vi "CSM - List Module Attributes.vi"(0 "CSM Name":string, 7 "Include Value? (F)":bool, 9 "Wait (5000 ms)":i32=5000, 11 "Error In":errorcluster caption="error in (no error)") -> (4 "CSM Name (Dup)":string, 6 "Attributes":string[](array[string]), 8 "Values":variant[](array[variant]), 10 "Waited (ms)":u32, 15 "error out":errorcluster)   [LabVIEW 2017, in "Communicable State Machine.lvlib"]
doc: "Lists all attribute names of the specified module. If the CSM module does not exist, this VI waits for the specified timeout duration. If the timeout is exceeded, this VI returns a timeout error.\n\n\n> [!NOTE] <b>CSM Module Attributes</b>\n>\n> CSM module attributes are a data area that can store module configuration and status, accessed by name. CSM module attributes can be used in the following scenarios:\n> - Providing a way to access and modify configuration and status information without messages. For example, a \"Connected\" attribute in a TCP module indicating whether a connection is established is more convenient to access directly.\n> - Nodes running in advanced modes, such as Worker Mode and Chain of Responsibility Mode, share the same data area, which is used for sharing data between modules.\n\n\n<b>Reference Example</b>: `[CSM-Example]\\0. Base Concepts\\6. Module Attributes.vi`.\n\n-- <b>Controls</b> --\n- <b>CSM Name</b>: CSM module name.\n- <b>Include Value? (F)</b>: Whether to include attribute values. The default is FALSE, which specifies to not include attribute values.\n- <b>Wait (5000 ms)</b>: Timeout duration for waiting module to be alive. The default is 5000 ms.\n\n-- <b>Indicators</b> --\n- <b>CSM Name (Dup)</b>: A copy of the input CSM module name.\n- <b>Attributes</b>: List of attribute names.\n- <b>Values</b>: List of attribute values.\n- <b>Waited (ms)</b>: Time elapsed while waiting."
uses:
  Communicable State Machine.lvlib
  _Support/CSMQ/_CSMOFGV(lvlibp).vi
  CSM - Wait for Module to Be Alive.vi
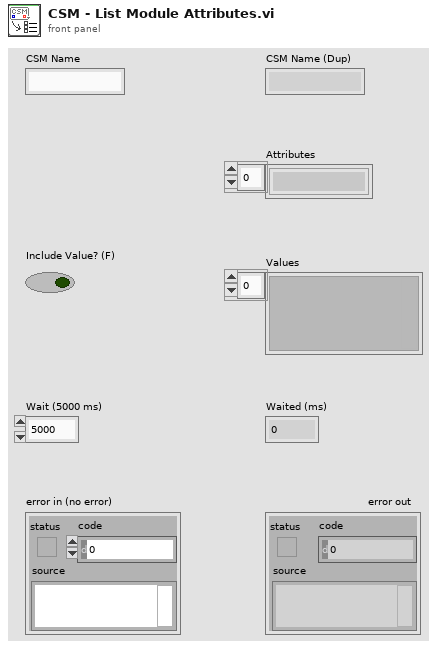
[diagram p1: front panel]
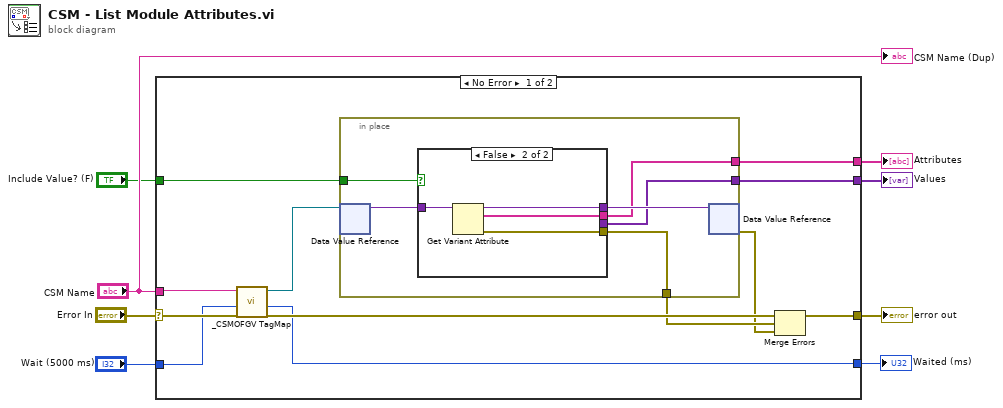
[diagram p0: block diagram]
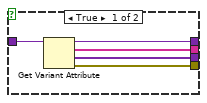
[diagram p2: hidden frame]
diagram:
  n1 = case shown="No Error" "Error In" {
    selector: "Error In" -> [w20 w36]
    tunnel: [w17 w36] -> w7
    tunnel: "CSM Name" -> [w11 _]
    tunnel: [w14 _] -> w5
    tunnel: [w13 _] -> w4
    tunnel: "Include Value? (F)" -> [w12 _]
    tunnel: "Wait (5000 ms)" -> [w10 _]
    tunnel: [w9 _] -> w1
    frame No Error {
      n2 = call "_CSMOFGV TagMap.vi"("error in (no error)"=w20, "Wait (5000 ms)"=w10, "CSM Name"=w11) -> ("error out"=w19:errorcluster, "Waited (ms)"=w9:u32, "TagMap"=w18:refnum<data-value>)  [unwired: 6 in]
      n3 = in-place {
        in-place-border: [w24] -> w16
        in-place-border: [w23] -> w14
        in-place-border: [w22] -> w13
        in-place-border: w12 -> [w21]
        n4 = in-place-dvr #1(w18) -> (w26:variant)  [unwired: 1 out]
        n5 = case shown="False" w21 {
          tunnel: w26 -> [w31 w35]
          tunnel: [w30 w34] -> w25
          tunnel: [w29 w33] -> w24
          tunnel: [w28 w32] -> w23
          tunnel: [w27 _] -> w22
          frame True {
            n6 = Get Variant Attribute(Variant=w31) -> (duplicate Variant=w30:variant, names=w28:string[], values=w27:variant[], error out=w29:errorcluster)  [unwired: 3 in]
          }
          frame False {
            n7 = Get Variant Attribute(Variant=w35) -> (duplicate Variant=w34:variant, names=w32:string[], error out=w33:errorcluster)  [unwired: 3 in, 1 out]
          }
        }
        n8 = in-place-dvr #1(w25) -> (w15:errorcluster)  [unwired: 1 out]
      }
      n9 = Merge Errors(w19, w16, w15) -> (w17:errorcluster)
    }
    frame Error {
    }
  }
  "error out" <- w7
  "Attributes" <- w5
  "Values" <- w4
  "Waited (ms)" <- w1
  "CSM Name (Dup)" <- "CSM Name"
